vi "Interpolate 1D Array RT Driver VI.vi"(7 "Operation":T4, 11 "Device Reference in":T5 format="%.0x") -> (0 "Error Code":i32)   [LabVIEW 2011, in "Interpolate 1D Array Custom Device.lvlib"]
uses:
  Interpolate 1D Array Custom Device.lvlib
  <vilib>/NI Veristand/Custom Device API/Custom Device Item Ref.ctl
  <vilib>/NI Veristand/Custom Device API/Model Interface Driver VI Operation.ctl
  Main Cluster Control.ctl
  <vilib>/NI Veristand/Custom Device API/Data Reference.ctl
  Interpolate Options.ctl
  Global Property Names.vi
  <vilib>/NI Veristand/Custom Device API/Get Item Property (Variant).vi
  <vilib>/NI Veristand/Custom Device API/Global Data Refs.vi
  <vilib>/NI Veristand/Custom Device API/Custom Device API.lvlib
  <vilib>/gmath/NI_Gmath.lvlib
panel:
  in  "cluster":T1={"Input Values"=[], "Input Refs"=[], "Output Values"=[], "Output Refs"=[], "Interpolate Info"={"Y Values"=[], "X Values"=[], "Interpolate Options"={"method"=1, "ntimes"=1, "X is monotonic"=FALSE}}, "New Values FIFO"=refnum, "Command FIFO"=refnum} {"Interpolate Info"."Interpolate Options"."method" items=["nearest", "linear", "spline", "cubic Hermite", "Lagrange"]; "Input Refs" format="%.0x"; "Output Refs" format="%.0x"}
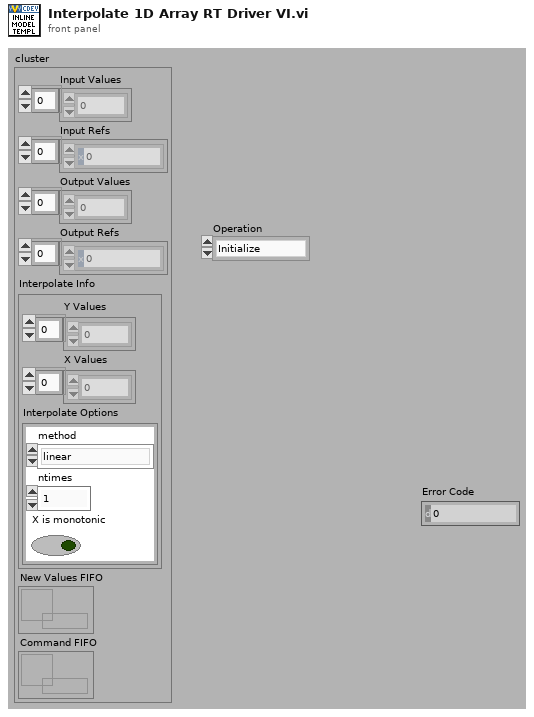
[diagram p1: front panel]
types:
  T1 = typedef "Interpolate 1D Array Custom Device.lvlib/Main Cluster Control.ctl" = cluster{"Input Values":dbl[], "Input Refs":T2[], "Output Values":dbl[], "Output Refs":T2[], "Interpolate Info":cluster{"Y Values":dbl[], "X Values":dbl[], "Interpolate Options":T3}, "New Values FIFO":refnum<k33>, "Command FIFO":refnum<k33>}
  T2 = typedef "Custom Device API.lvlib/Data Reference.ctl" = i32
  T3 = typedef "Interpolate 1D Array Custom Device.lvlib/Interpolate Options.ctl" = cluster{"method":i32, "ntimes":i32, "X is monotonic":bool}
  T4 = typedef "Custom Device API.lvlib/Model Interface Driver VI Operation.ctl" = enum16{"Initialize", "Start", "Execute Model", "Close"}
  T5 = typedef "Custom Device API.lvlib/Custom Device Item Ref.ctl" = u64
  T6 = cluster{"read mode":enum16{"polling", "blocking"}, "write mode":enum16{"polling", "blocking"}}
  T7 = cluster{"Y Values":dbl[], "X Values":dbl[], "Interpolate Options":T3}
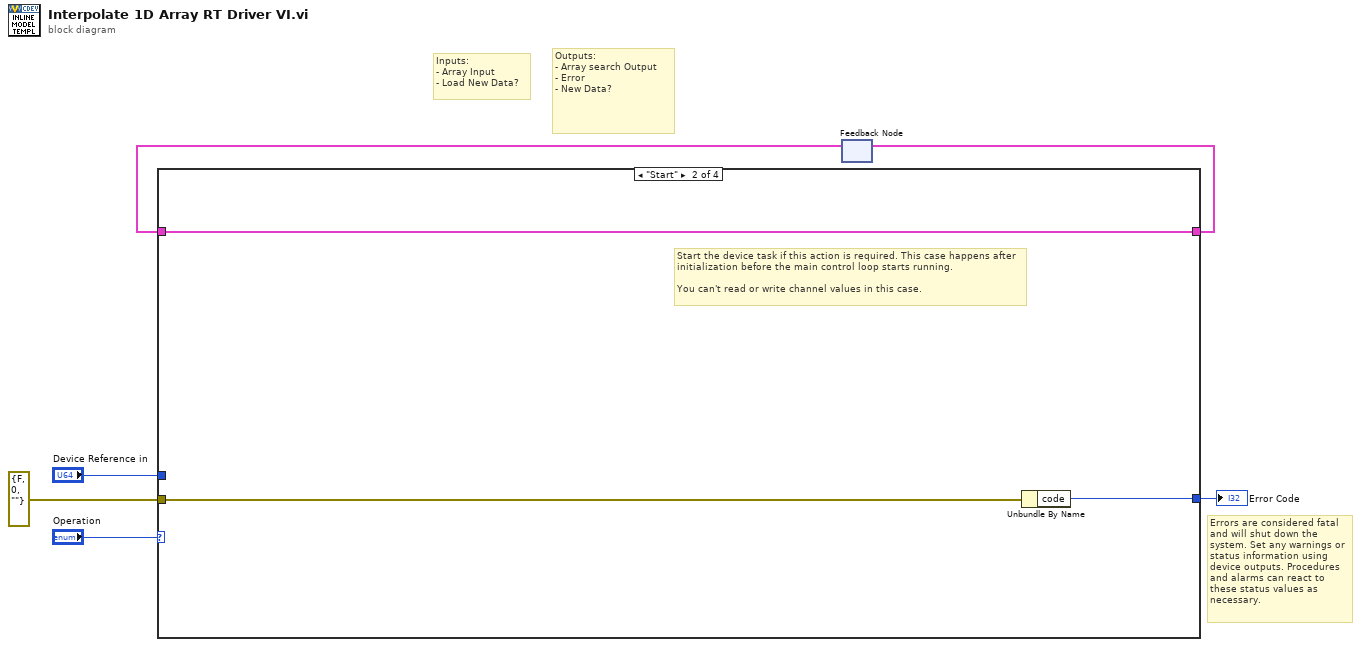
[diagram p0: block diagram]
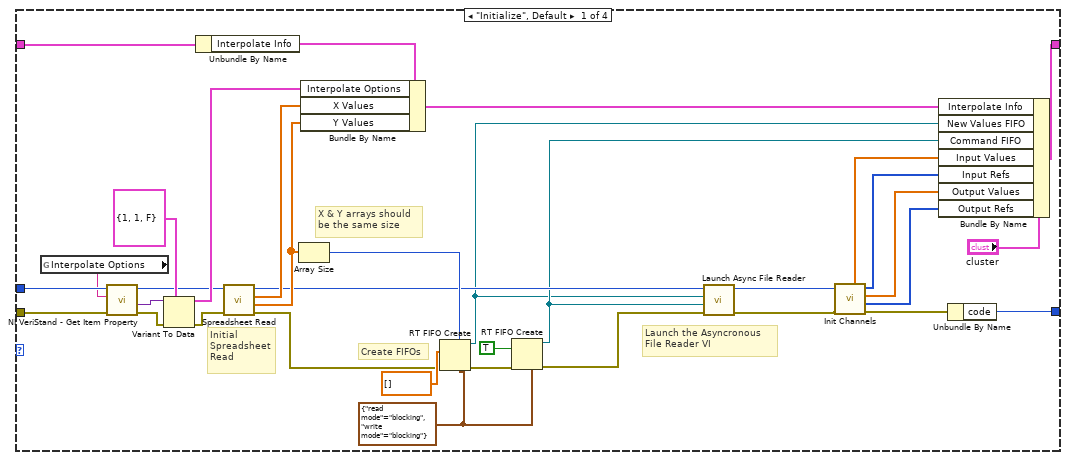
[diagram p2: hidden frame]
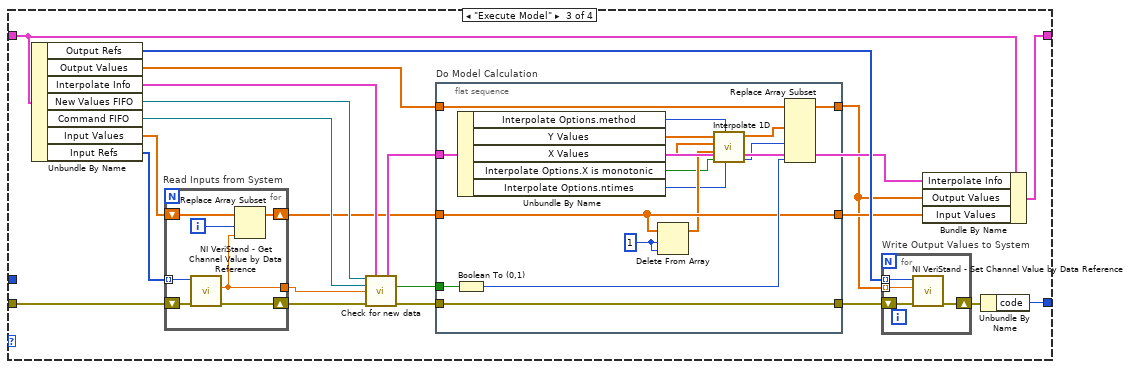
[diagram p3: hidden frame]
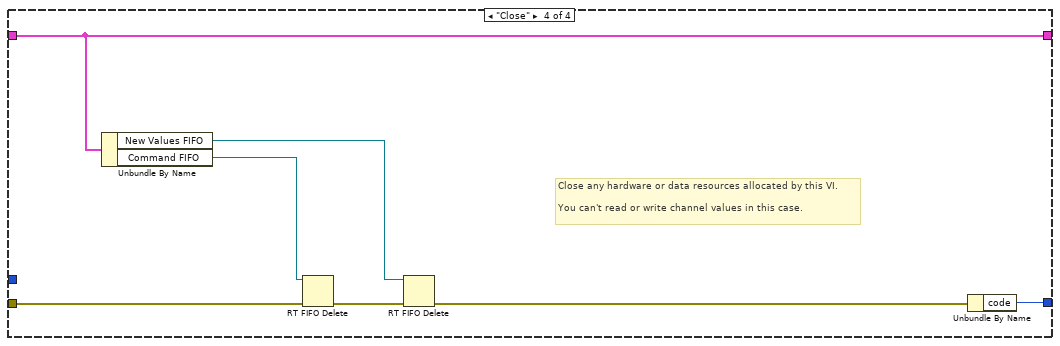
[diagram p4: hidden frame]
diagram:
  # "Outputs:\n- Array search Output\n- Error\n- New Data?"
  # "Inputs:\n- Array Input\n- Load New Data?"
  # "Errors are considered fatal and will shut down the system. Set any warnings or status information using device outputs. Procedures and alarms can react to these status values as necessary."
  n1 = feedback #1() -> (w4:T1)  [unwired: 1 out]
  n2 = case shown="\"Start\"" "Operation" {
    tunnel: [w40 w43 w60 w97] -> w5
    tunnel: w4 -> [w29 w43 w61 w97]
    tunnel: "Device Reference in" -> [w37 _ _ _]
    tunnel: [w39 w41 w57 w98] -> w2
    tunnel: errorcluster {"status"=FALSE, "code"=0, "source"=""} ("error in (no error)") -> [w36 w42 w62 w96]
    frame "Initialize", Default {
      w18 = T6 {"read mode"=enum."blocking", "write mode"=enum."blocking"} ("r/w modes (polling,polling)")
      # "Launch the Asyncronous\nFile Reader VI"
      # "Create FIFOs"
      # "Initial\nSpreadsheet\nRead"
      # "X & Y arrays should\nbe the same size"
      n3 = global read "Global Property Names.vi" "Interpolate Options"() -> (w35:string)
      n4 = call-poly <vilib>:"NI VeriStand - Get Item Property.vi"("error in (no error)"=w36, "Property Name"=w35, "Item Ref in"=w37) -> ("error out"=w32:errorcluster, "Value"=w34:variant, "Item Ref out"=w27:T5)  [unwired: 5 in, 1 out]
      n5 = Variant To Data(error in=w32, type=T3 {"method"=1, "ntimes"=1, "X is monotonic"=FALSE} ("Interpolate Options"), Variant=w34) -> (data=w31:T3, error out=w26:errorcluster)
      n6 = Unbundle By Name(w29) -> ("Interpolate Info"=w28:T7)
      n7 = call "Spreadsheet Read.vi"("error in (no error)"=w26, "Device Reference in"=w27) -> ("error out"=w13:errorcluster, "Y Array"=w14:dbl[], "X Array"=w15:dbl[], "Device Reference Out"=w11:T5)  [unwired: 6 in]
      n8 = Array Size(array=w14) -> (size(s)=w16:i32)
      n9 = Bundle By Name(cluster=w28, "Interpolate Options"=w31, "X Values"=w15, "Y Values"=w14) -> (w30:T7)
      n10 = RT FIFO Create(1:dbl[] [] ("Y Array"), 3:w13, 6:w16, 7:w18) -> (8:w7:refnum<k33>, 11:w19:errorcluster)  [unwired: 4 in, 1 out]
      n11 = RT FIFO Create(1:TRUE, 3:w19, 7:w18) -> (8:w8:refnum<k33>, 11:w12:errorcluster)  [unwired: 5 in, 1 out]
      n12 = call "Launch Async File Reader.vi"("error in (no error)"=w12, "Command FIFO"=w8, "New Values FIFO"=w7, "Device Reference in"=w11) -> ("error out"=w9:errorcluster, "Device Reference Out"=w10:T5)  [unwired: 6 in]
      n13 = call "Init Channels.vi"("error in (no error)"=w9, "Device Item Ref In"=w10) -> ("error out"=w20:errorcluster, "Output Refs"=w21:T2[], "Output Values"=w22:dbl[], "Input Refs"=w23:T2[], "Input Values"=w24:dbl[])  [unwired: 5 in]
      n14 = Bundle By Name(cluster="cluster", "Interpolate Info"=w30, "New Values FIFO"=w7, "Command FIFO"=w8, "Input Values"=w24, "Input Refs"=w23, "Output Values"=w22, "Output Refs"=w21) -> (w40:T1)
      n15 = Unbundle By Name(w20) -> ("code"=w39:i32)
    }
    frame "Start" {
      # "Start the device task if this action is required. This case happens after initialization before the main control loop starts running.\n\nYou can't read or write channel values in this case."
      n16 = Unbundle By Name(w42) -> ("code"=w41:i32)
    }
    frame "Execute Model" {
      n17 = Unbundle By Name(w61) -> ("Output Refs"=w59:T2[], "Output Values"=w56:dbl[], "Interpolate Info"=w54:T7, "New Values FIFO"=w52:refnum<k33>, "Command FIFO"=w51:refnum<k33>, "Input Values"=w64:dbl[], "Input Refs"=w63:T2[])
      n18 = for "Read Inputs from System" {
        shift-right: [w86] -> w49
        shift-left: w62 -> [w91]
        tunnel: w63 -> [w90] mode=indexing
        shift-right: [w88] -> w44
        shift-left: w64 -> [w89]
        tunnel: [w85] -> w50
        i -> [w87]
        n19 = call <vilib>:"NI VeriStand - Get Channel Value by Data Reference.vi"("error in (no error)"=w91, "Data Reference in"=w90) -> ("error out"=w86:errorcluster, "Value"=w85:dbl)  [unwired: 8 out]
        n20 = Replace Array Subset(array=w89, new element=w85, index=w87) -> (w88:dbl[])
      }
      n21 = call "Check for new data.vi"("New Value FIFO"=w52, "Interpolate Info In"=w54, "Command FIFO"=w51, "Load New Data?"=w50, "error in (no error)"=w49) -> ("Interpolate Info Out"=w53:T7, "New Data Ready?"=w47:bool, "error out"=w48:errorcluster)  [unwired: 8 in]
      n22 = flat-sequence "Do Model Calculation" {
        tunnel: w48 -> [w84]
        tunnel: w56 -> [w83]
        tunnel: [w82] -> w46
        tunnel: [w84] -> w45
        tunnel: w53 -> [w81]
        tunnel: w44 -> [w77]
        tunnel: [w77] -> w55
        tunnel: w47 -> [w80]
        frame #0 {
          w78 = 1 ("length")
          n23 = Boolean To (0,1)(Boolean=w80) -> (0, 1=w79:i16)
          n24 = Unbundle By Name(w81) -> ("Interpolate Options.method"=w76:i32, "Y Values"=w75:dbl[], "X Values"=w74:dbl[], "Interpolate Options.X is monotonic"=w72:bool, "Interpolate Options.ntimes"=w71:i32)
          n25 = Delete From Array(array=w77, length=w78, index=w78) -> (array with subset deleted=w73:dbl[])  [unwired: 1 out]
          n26 = call <vilib>:"Interpolate 1D.vi"("ntimes"=w71, "method"=w76, "X is monotonic"=w72, "xi"=w73, "X"=w74, "Y"=w75) -> ("error"=w70:i32, "yi"=w69:dbl[])  [unwired: 3 in, 1 out]
          n27 = Replace Array Subset(array=w83, new element #1=w69, new element #2=w70, new element #3=w79) -> (w82:dbl[])  [unwired: 3 in]
        }
      }
      n28 = for "Write Output Values to System" {
        shift-right: [w67] -> w58
        shift-left: w45 -> [w68]
        tunnel: w46 -> [w66] mode=indexing
        tunnel: w59 -> [w65] mode=indexing
        n29 = call <vilib>:"NI VeriStand - Set Channel Value by Data Reference.vi"("error in (no error)"=w68, "Value"=w66, "Data Reference in"=w65) -> ("error out"=w67:errorcluster)  [unwired: 8 out]
      }
      n30 = Bundle By Name(cluster=w61, "Interpolate Info"=w53, "Output Values"=w46, "Input Values"=w55) -> (w60:T1)
      n31 = Unbundle By Name(w58) -> ("code"=w57:i32)
    }
    frame "Close" {
      # "Close any hardware or data resources allocated by this VI.\n\nYou can't read or write channel values in this case."
      n32 = Unbundle By Name(w97) -> ("New Values FIFO"=w92:refnum<k33>, "Command FIFO"=w93:refnum<k33>)
      n33 = RT FIFO Delete(0:w93, 3:w96) -> (11:w94:errorcluster)  [unwired: 1 in]
      n34 = RT FIFO Delete(0:w92, 3:w94) -> (11:w95:errorcluster)  [unwired: 1 in]
      n35 = Unbundle By Name(w95) -> ("code"=w98:i32)
    }
  }
  "Error Code" <- w2
  n36 = feedback-in #1(w5) -> ()
